vi "Using a previously exported configuration - part 2.vi"(8 "error in (no error)":errorcluster, 10 "configuration file path":path, 11 "target in":refnum<k24>) -> (0 "error out":errorcluster)   [LabVIEW 2019]
uses:
  NationalInstruments.VeriStand.SystemDefinitionAPI
  <vilib>/addons/VeriStand Custom Device Scripting APIs/Instrument Addon/API/TypeDefs/Single Channel Type Cast Settings.ctl
  <vilib>/addons/VeriStand Custom Device Scripting APIs/Instrument Addon/Shared Directory/Type Cast Type.ctl
  <vilib>/addons/VeriStand Custom Device Scripting APIs/Instrument Addon/Shared Directory/Endian.ctl
  <vilib>/addons/VeriStand Custom Device Scripting APIs/Instrument Addon/API/TypeDefs/ByteCount Response Settings.ctl
  <vilib>/addons/VeriStand Custom Device Scripting APIs/Instrument Addon/API/TypeDefs/Linked Channel.ctl
  <vilib>/NI VeriStand/Custom Device API/Custom Device Item Ref.ctl
  <vilib>/addons/VeriStand Custom Device Scripting APIs/Instrument Addon/API/Channels/Create Data Channel - Single Channel - Type Cast.vi
  <vilib>/addons/VeriStand Custom Device Scripting APIs/Instrument Addon/API/Messages/Configure Response - Byte Count.vi
  <vilib>/addons/VeriStand Custom Device Scripting APIs/Instrument Addon/API/Instrument Addon Scripting API.lvlib
  <vilib>/NI VeriStand/Custom Device API/Custom Device API.lvlib
  <vilib>/addons/VeriStand Custom Device Scripting APIs/Instrument Addon/Shared Directory/Instrument Addon Shared.lvlib
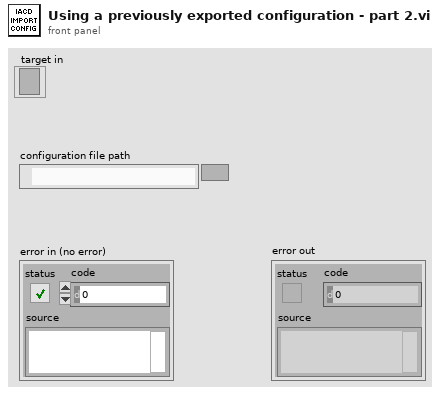
[diagram p1: front panel]
types:
  T1 = typedef "Instrument Addon Scripting API.lvlib/Linked Channel.ctl" = cluster{"Variable Name":string, "Channel Refnum":T2}
  T2 = typedef "Custom Device API.lvlib/Custom Device Item Ref.ctl" = u64
  T3 = typedef "Instrument Addon Scripting API.lvlib/ByteCount Response Settings.ctl" = cluster{"Response Format":string, "Linked Channels":T1[], "Byte Count":i32, "Use Byte Count channel":bool, "Channel Refnum":T2}
  T4 = typedef "Instrument Addon Scripting API.lvlib/Single Channel Type Cast Settings.ctl" = cluster{"Default Value":dbl, "Units":string, "Type":T5, "Endian":T6}
  T5 = typedef "Instrument Addon Shared.lvlib/Type Cast Type.ctl" = enum16{"DBL", "SGL", "U64", "U32", "U16", "U8", "I64", "I32", "I16", "I8"}
  T6 = typedef "Instrument Addon Shared.lvlib/Endian.ctl" = enum16{"Native", "Little", "Big"}
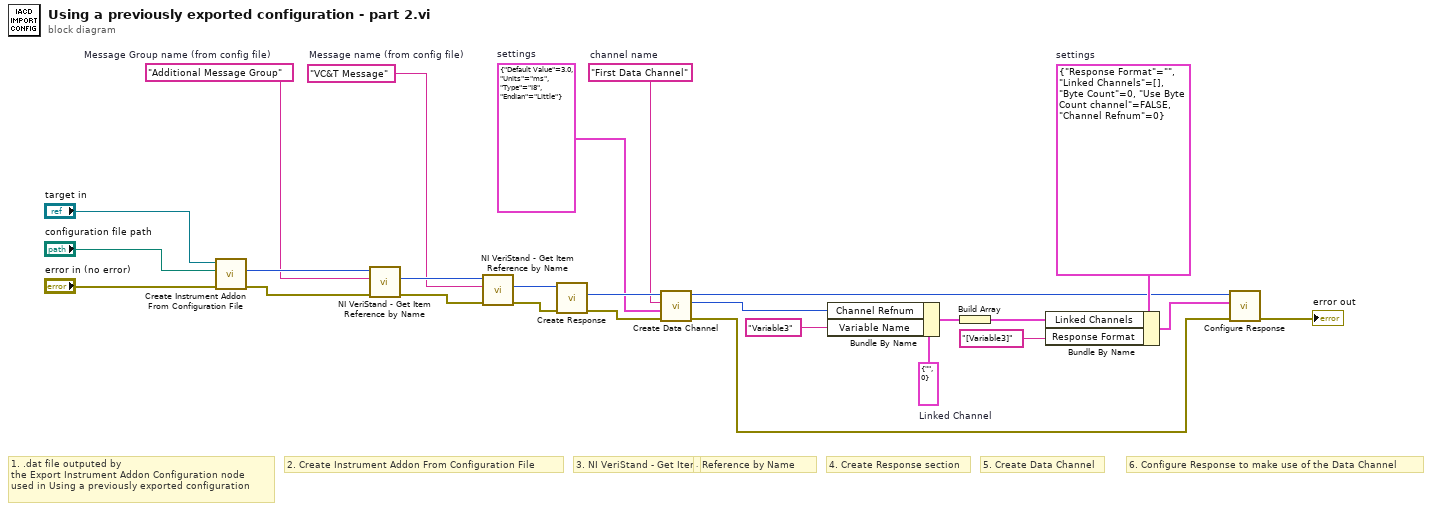
[diagram p0: block diagram]
diagram:
  w7 = T1 {"Variable Name"="", "Channel Refnum"=0}  # Linked Channel
  w8 = T3 {"Response Format"="", "Linked Channels"=[], "Byte Count"=0, "Use Byte Count channel"=FALSE, "Channel Refnum"=0}  # settings
  w13 = T4 {"Default Value"=3.0, "Units"="ms", "Type"=enum."I8", "Endian"=enum."Little"}  # settings
  w14 = "First Data Channel"  # channel name
  w19 = "VC&T Message"  # Message name (from config file)
  w22 = "Additional Message Group"  # Message Group name (from config file)
  # "6. Configure Response to make use of the Data Channel"
  # "5. Create Data Channel"
  # "4. Create Response section"
  # "2. Create Instrument Addon From Configuration File"
  # "1. .dat file outputed by\nthe Export Instrument Addon Configuration node\nused in Using a previously exported configuration"
  # "3. NI VeriStand - Get Item Reference by Name"
  # "."
  n1 = call <vilib>:"Create Instrument Addon From Configuration File.vi"("error in (no error)"="error in (no error)", "configuration file path"="configuration file path", "target in"="target in") -> ("error out"=w21:errorcluster, "instrument addon refnum"=w23:T2)  [unwired: 6 in, 1 out]
  n2 = call <vilib>:"NI VeriStand - Get Item Reference by Name.vi"("error in (no error)"=w21, "Item Name"=w22, "Parent Ref in"=w23) -> ("error out"=w18:errorcluster, "Item Ref"=w20:T2)  [unwired: 5 in, 2 out]
  n3 = call <vilib>:"NI VeriStand - Get Item Reference by Name.vi"("error in (no error)"=w18, "Item Name"=w19, "Parent Ref in"=w20) -> ("error out"=w16:errorcluster, "Item Ref"=w17:T2)  [unwired: 5 in, 2 out]
  n4 = call <vilib>:"Create Response.vi"("error in (no error)"=w16, "message refnum in"=w17) -> ("error out"=w12:errorcluster, "response refnum"=w15:T2)  [unwired: 7 in, 1 out]
  n5 = call-poly <vilib>:"Create Data Channel.vi"("error in (no error)"=w12, "settings"=w13, "channel name"=w14, "response refnum in"=w15) -> ("error out"=w2:errorcluster, "channel refnum"=w9:T2, "response refnum out"=w4:T2)  [unwired: 5 in]
  n6 = Bundle By Name(cluster=w7, "Channel Refnum"=w9, "Variable Name"="Variable3") -> (w10:T1)
  n7 = Build Array(w10) -> (w6:T1[])
  n8 = Bundle By Name(cluster=w8, "Linked Channels"=w6, "Response Format"="[Variable3]" ("Command Format")) -> (w5:T3)
  n9 = call-poly <vilib>:"Configure Response.vi"("error in (no error)"=w2, "settings"=w5, "response refnum in"=w4) -> ("error out"=→"error out":errorcluster)  [unwired: 7 in, 1 out]
